vi "PaiedTunnels - Connect Wire.vi"(8 "Error in":errorcluster caption="Error in (no error)", 10 "index(-1 for all)":i32=-1, 11 "PaiedTunnels":cluster{"Left":refnum<vi>, "Right":refnum<vi>}) -> (0 "Error out":errorcluster, 3 "PaiedTunnels":cluster{"Left":refnum<vi>, "Right":refnum<vi>})   [LabVIEW 2017, in "CSM-Helper.lvclass"]
uses:
  CSM-Helper.lvclass
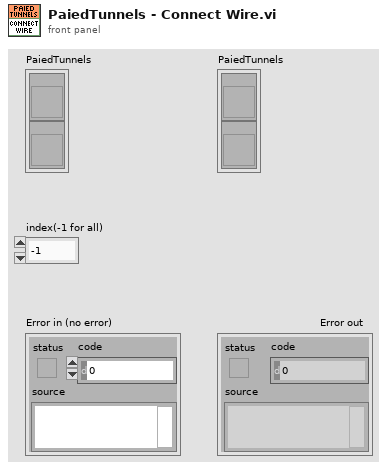
[diagram p1: front panel]
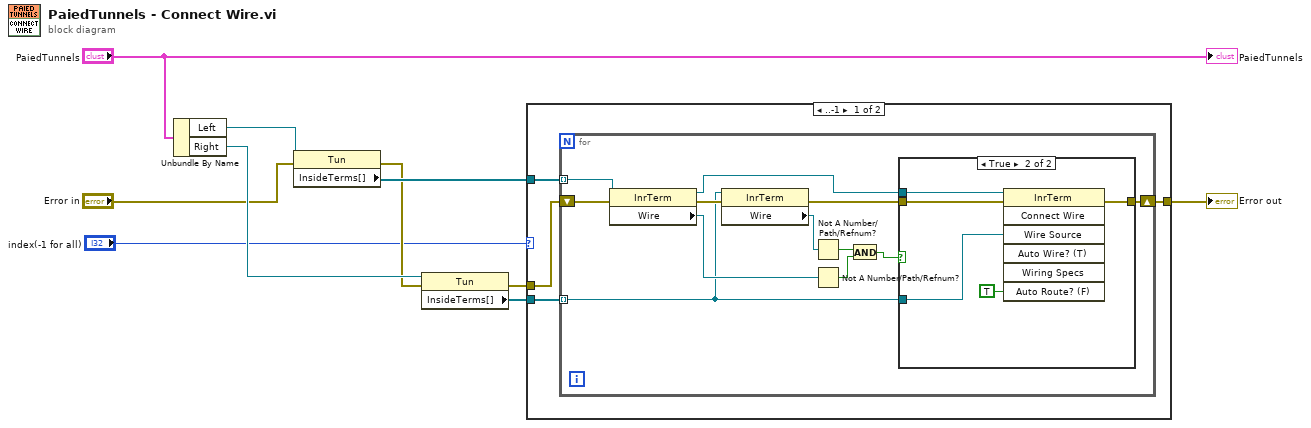
[diagram p0: block diagram]
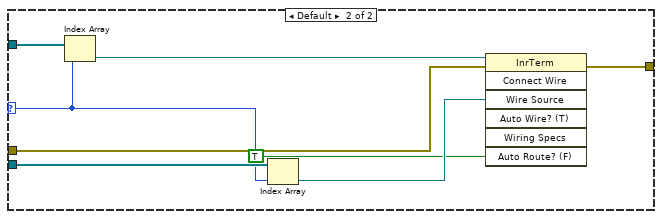
[diagram p3: hidden frame]
diagram:
  n1 = Unbundle By Name("PaiedTunnels") -> ("Left"=w10:refnum<vi>, "Right"=w9:refnum<vi>)
  n2 = property on="Property Node" class="Tun"(reference=w10, error in="Error in") -> (error out=w6:errorcluster, "InsideTerms[]"=w8:refnum<vi>[])  [unwired: 1 out]
  n3 = property on="Property Node" class="Tun"(reference=w9, error in=w6) -> (error out=w5:errorcluster, "InsideTerms[]"=w7:refnum<vi>[])  [unwired: 1 out]
  n4 = case shown="..-1" "index(-1 for all)" {
    selector: "index(-1 for all)" -> [_ w33]
    tunnel: w8 -> [w14 w40]
    tunnel: w7 -> [w13 w39]
    tunnel: w5 -> [w12 w35]
    tunnel: [w11 w34] -> w4
    frame ..-1 {
      n5 = for {
        tunnel: w14 -> [w25] mode=indexing
        tunnel: w13 -> [w16] mode=indexing
        shift-right: [w26] -> w11
        shift-left: w12 -> [w24]
        n6 = property on="Property Node" class="InrTerm"(reference=w25, error in=w24) -> (reference out=w15:refnum<vi>, error out=w23:errorcluster, "Wire"=w20:refnum<vi>)
        n7 = property on="Property Node" class="InrTerm"(reference=w16, error in=w23) -> (error out=w22:errorcluster, "Wire"=w21:refnum<vi>)  [unwired: 1 out]
        n8 = Not A Number/Path/Refnum?(number/path/refnum=w21) -> (NaN/Path/Refnum?=w19:bool)
        n9 = Not A Number/Path/Refnum?(number/path/refnum=w20) -> (NaN/Path/Refnum?=w18:bool)
        n10 = And(x=w19, y=w18) -> (x .and. y?=w17:bool)
        n11 = case shown="True" w17 {
          tunnel: [w27 w31] -> w26
          tunnel: w16 -> [_ w30]
          tunnel: w22 -> [w27 w29]
          tunnel: w15 -> [_ w28]
          frame False {
          }
          frame True {
            n12 = invoke on="Invoke Node" class="InrTerm" method="Connect Wire"(reference=w28, error in=w29, "Wire Source"=w30, "Auto Route? (F)"=TRUE) -> (error out=w31:errorcluster)  [unwired: 3 in, 6 out]
          }
        }
      }
    }
    frame Default {
      n13 = Index Array(array=w40, index=w33) -> (element=w38:refnum<vi>)
      n14 = Index Array(array=w39, index=w33) -> (element=w37:refnum<vi>)
      n15 = invoke on="Invoke Node" class="InrTerm" method="Connect Wire"(reference=w38, error in=w35, "Wire Source"=w37, "Auto Route? (F)"=TRUE) -> (error out=w34:errorcluster)  [unwired: 3 in, 6 out]
    }
  }
  "Error out" <- w4
  "PaiedTunnels" <- "PaiedTunnels"
